vi "Tolerance(SubVI).vi"(4 "Tolerance":T1, 5 "x*y":dbl) -> (1 "x-y":dbl, 2 "x+y":dbl)   [LabVIEW 2018]
uses:
  Tolerance.ctl
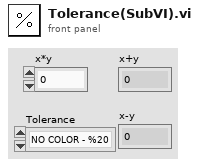
[diagram p1: front panel]
types:
  T1 = typedef "Tolerance.ctl" = enum16{"NO COLOR - %20", "Brown - %1", "Red - %2", "Orange - %3", "Yellow - %4", "Green - %0,5", "Blue - %0,25", "Violet - %0,10", "Grey - %0,05", "Silver x - %10", "Gold x - %5"}
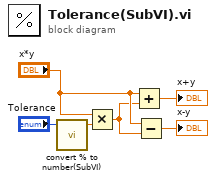
[diagram p0: block diagram]
diagram:
  n1 = call "convert % to number(SubVI).vi"("Tolerance"="Tolerance") -> ("Numeric"=w2:dbl)  [unwired: 4 in]
  n2 = Multiply(x="x*y", y=w2) -> (x*y=w3:dbl)
  n3 = Add(x="x*y", y=w3) -> (x+y=→"x+y":dbl)
  n4 = Subtract(x="x*y", y=w3) -> (x-y=→"x-y":dbl)
